vi "Analog Output DAQ Engine.vi"(8 "error in":errorcluster, 10 "DAQ Engine":refnum<notifier>, 11 "Sequence Context In":refnum<k7>) -> (0 "error out":errorcluster)   [LabVIEW 2023, in "LTT_TeststandSteptypes.lvlib"]
uses:
  LTT_TeststandSteptypes.lvlib
  HardwareAbstractionLayer_LVOOP/Main/Class Ref.ctl
  HardwareAbstractionLayer_LVOOP/DMM/DMM.lvclass
  HardwareAbstractionLayer_LVOOP/Function Generator/Function Generator.lvclass
  HardwareAbstractionLayer_LVOOP/Oscilloscope/Oscilloscope.lvclass
  HardwareAbstractionLayer_LVOOP/PowerSupply/PowerSupply.lvclass
  HardwareAbstractionLayer_LVOOP/Teststand/Teststand.lvclass
  HardwareAbstractionLayer_LVOOP/Analog Output/AO/AO.lvclass
  HardwareAbstractionLayer_LVOOP/Analog Input/AI/AI.lvclass
  HardwareAbstractionLayer_LVOOP/Database/Database.lvclass
  HardwareAbstractionLayer_LVOOP/Digital Output/DO_class/DO.lvclass
  HardwareAbstractionLayer_LVOOP/Digital Input/DI_class/DI.lvclass
  HardwareAbstractionLayer_LVOOP/PWM Output/PWM Output_class/PWM Output.lvclass
  HardwareAbstractionLayer_LVOOP/PWM Input/PWM Input_class/PWM Input.lvclass
  HardwareAbstractionLayer_LVOOP/NI Switch/NISwitch_class/NISwitch.lvclass
  HardwareAbstractionLayer_LVOOP/Modbus/Modbus_class/Modbus.lvclass
  HardwareAbstractionLayer_LVOOP/CAN/CAN Lib/CAN_class/CAN.lvclass
  HardwareAbstractionLayer_LVOOP/Analog Output/NI Analog Output/NI Analog Output.lvclass
  D:/eDCU LTT/VT LTT Project/Source Code/HardwareAbstractionLayer_LVOOP/Analog Output/AO/AO.lvclass
  HardwareAbstractionLayer_LVOOP/Main/Class Options.ctl
  <vilib>/Utility/error.llb/DialogType.ctl
  HardwareAbstractionLayer_LVOOP/Main/Main.lvclass
panel:
  in  "stop":bool
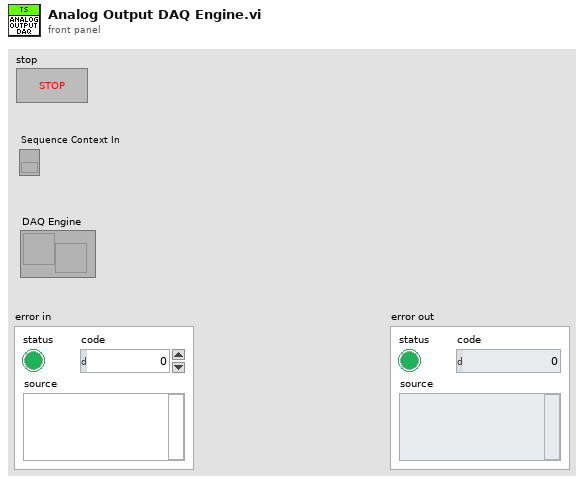
[diagram p1: front panel]
types:
  T1 = typedef "HardwareAbstractionLayer_LVOOP.lvlib/Main.lvclass/Class Ref.ctl" = cluster{"DMM":refnum<class "DMM.lvclass">, "Function Generator":refnum<class "Function Generator.lvclass">, "Oscilloscope":refnum<class "Oscilloscope.lvclass">, "PowerSupply":refnum<class "PowerSupply.lvclass">, "Teststand":refnum<class "Teststand.lvclass">, "AO":refnum<class "AO.lvclass">, "AI":refnum<class "AI.lvclass">, "Database":refnum<class "Database.lvclass">, "AO Waveform Generation":refnum<class "AO.lvclass">, "DO":refnum<class "DO.lvclass">, "DI":refnum<class "DI.lvclass">, "PWM Output":refnum<class "PWM Output.lvclass">, "PWM Input":refnum<class "PWM Input.lvclass">, "RelayOutput":refnum<class "NISwitch.lvclass">, "Modbus":refnum<class "Modbus.lvclass">, "CAN":refnum<class "CAN.lvclass">}
  T2 = typedef "HardwareAbstractionLayer_LVOOP.lvlib/Main.lvclass/Class Options.ctl" = enum16{"Init All Class", "Read All Class", "Write AI Class", "Write AO Class", "Write AO Waveform Generation", "Write DI Class", "Write DO Class", "Write PWM Input Class", "Write PWM Output Class", "Exit"}
  T3 = typedef "DialogType.ctl" = u16
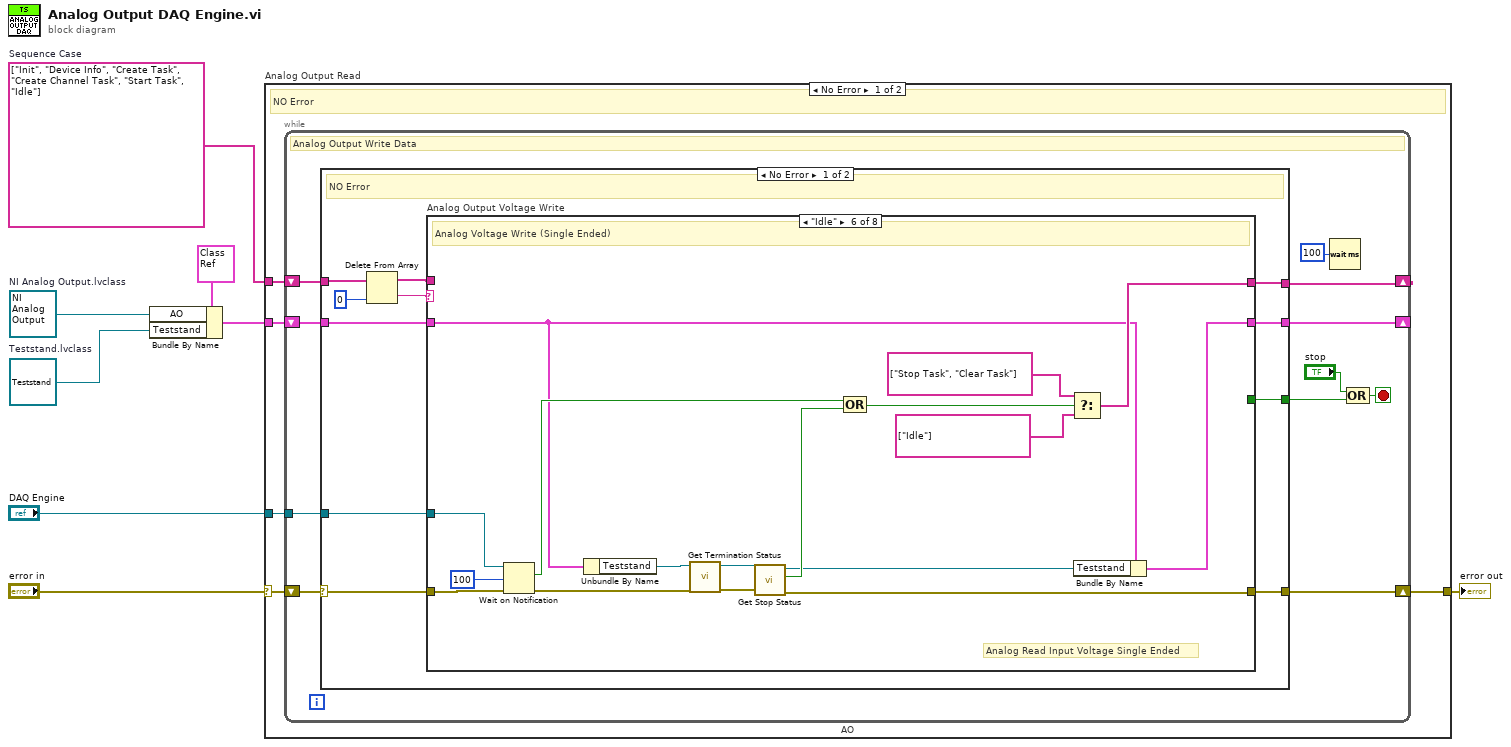
[diagram p0: block diagram]
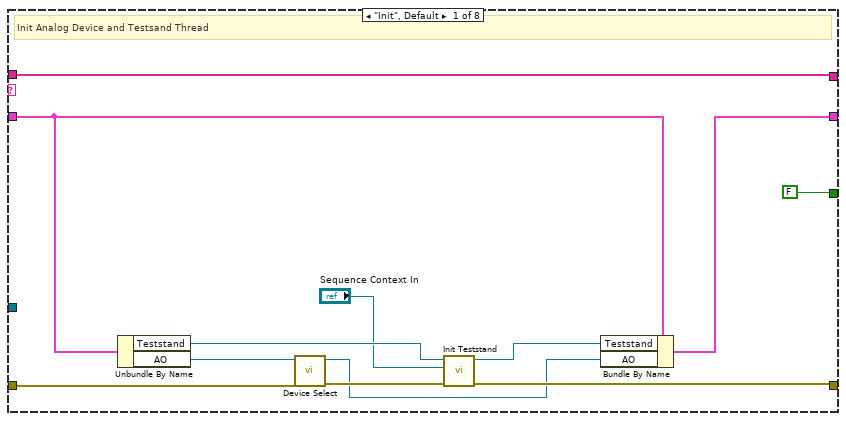
[diagram p2: hidden frame]
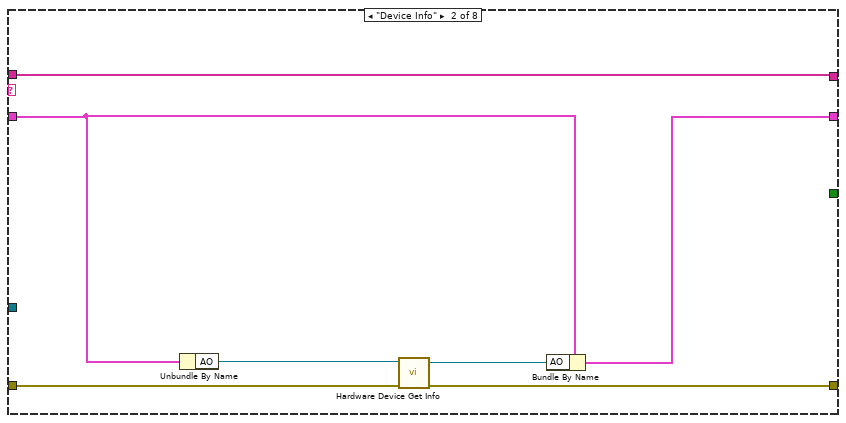
[diagram p3: hidden frame]
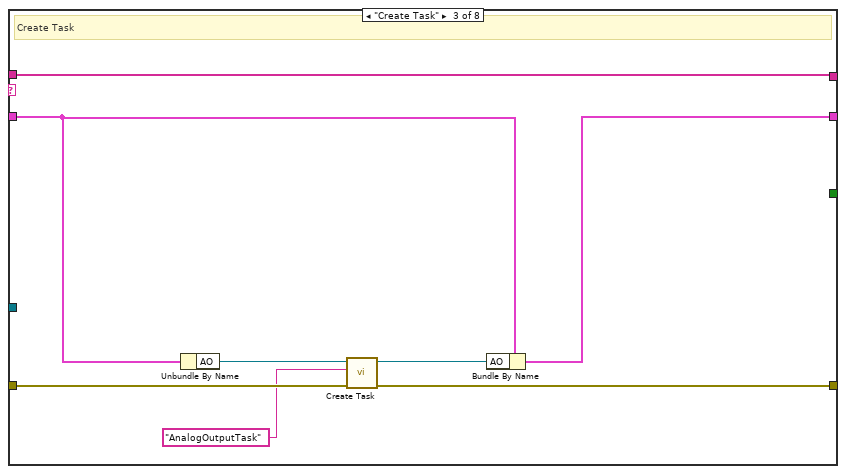
[diagram p4: hidden frame]
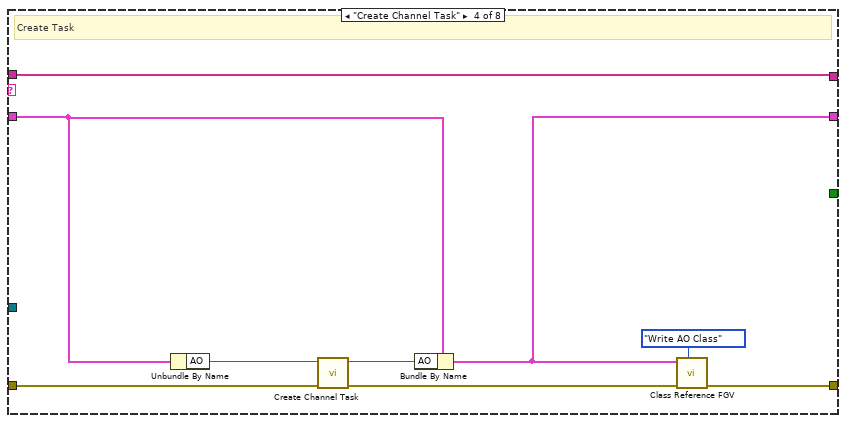
[diagram p5: hidden frame]
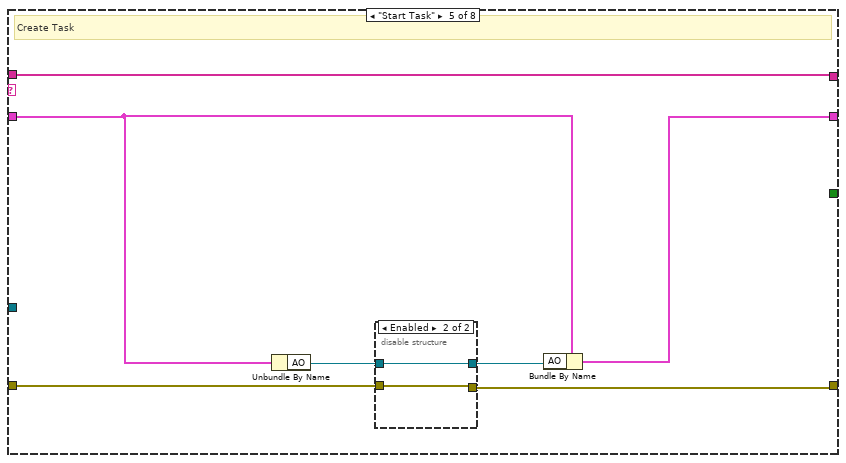
[diagram p6: hidden frame]
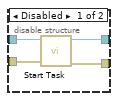
[diagram p7: hidden frame]
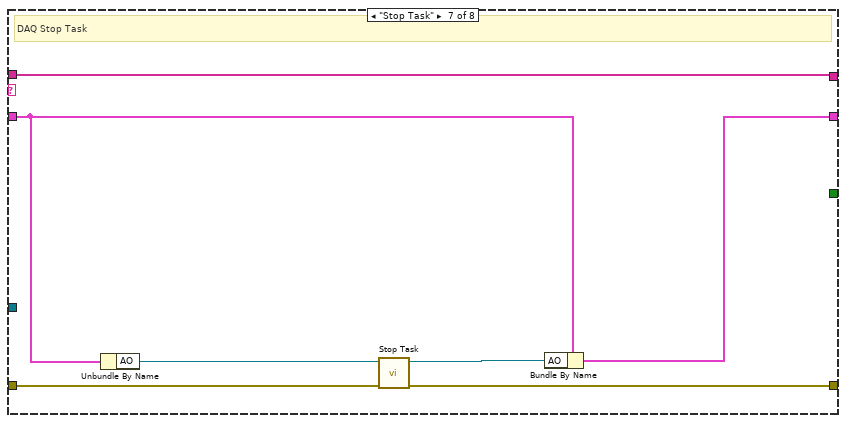
[diagram p8: hidden frame]
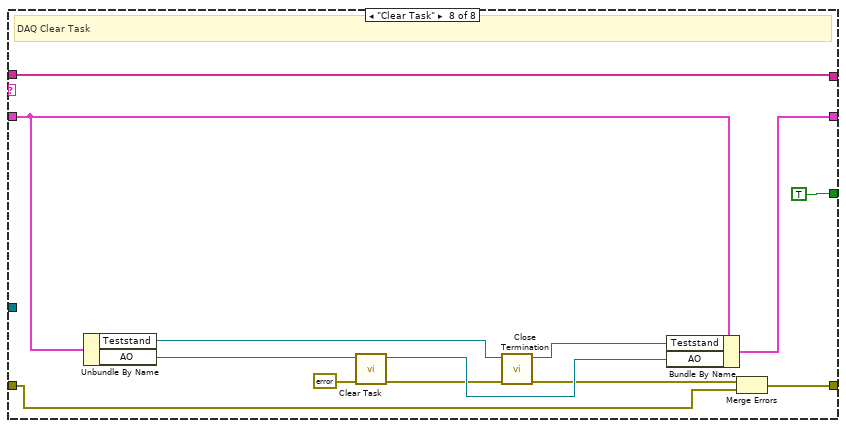
[diagram p9: hidden frame]
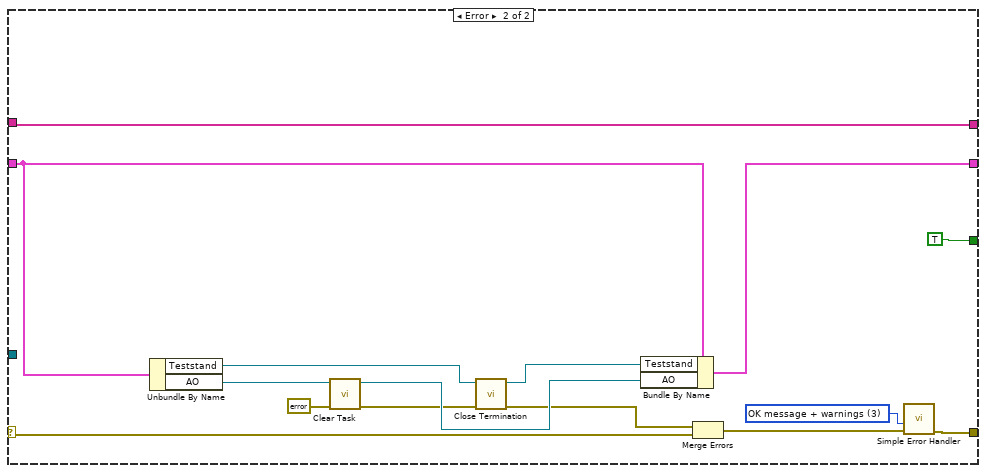
[diagram p10: hidden frame]
diagram:
  w1 = refnum<class "Teststand.lvclass"> refnum  # Teststand.lvclass
  w3 = refnum<class "NI Analog Output.lvclass"> refnum  # NI Analog Output.lvclass
  w4 = string[] ["Init", "Device Info", "Create Task", "Create Channel Task", "Start Task", "Idle"]  # Sequence Case
  n1 = Bundle By Name(cluster=T1 {"DMM"=refnum, "Function Generator"=refnum, "Oscilloscope"=refnum, "PowerSupply"=refnum, "Teststand"=refnum, "AO"=refnum, "AI"=refnum, "Database"=refnum, "AO Waveform Generation"=refnum, "DO"=refnum, "DI"=refnum, "PWM Output"=refnum, "PWM Input"=refnum, "RelayOutput"=refnum, "Modbus"=refnum, "CAN"=refnum} ("Class Cluster"), "AO"=w3, "Teststand"=w1) -> (w5:T1)
  n2 = case "Analog Output Read" shown="No Error" "error in" {
    selector: "error in" -> [w13 w137]
    tunnel: [w12 w137] -> w7
    tunnel: w5 -> [w11 _]
    tunnel: w4 -> [w10 _]
    tunnel: "DAQ Engine" -> [w9 _]
    frame No Error {
      # "NO Error"
      n3 = while "AO" {
        shift-right: [w23] -> w12
        shift-left: w13 -> [w24]
        shift-right: [w21] -> _
        shift-left: w11 -> [w22]
        shift-right: [w19] -> _
        shift-left: w10 -> [w20]
        tunnel: w9 -> [w14]
        stop <- w16 stop-if-true
        # "Analog Output Write Data"
        n4 = case shown="No Error" w24 {
          selector: w24 -> [w35 w128]
          tunnel: [w34 w123] -> w23
          tunnel: w22 -> [w30 w126]
          tunnel: [w29 w127] -> w21
          tunnel: w20 -> [w33 w125]
          tunnel: [w27 w125] -> w19
          tunnel: [w26 TRUE] -> w15
          tunnel: w14 -> [w25 _]
          frame No Error {
            # "NO Error"
            n5 = Delete From Array(array=w33, index=0) -> (deleted portion=w32:string, array with subset deleted=w28:string[])  [unwired: 1 in]
            n6 = case "Analog Output Voltage Write" shown="\"Idle\"" w32 {
              tunnel: w35 -> [w43 w51 w59 w69 w75 w101 w105 w109]
              tunnel: [w38 w50 w58 w65 w73 w89 w104 w110] -> w34
              tunnel: w30 -> [w46 w53 w61 w70 w77 w87 w107 w120]
              tunnel: [w45 w52 w60 w63 w76 w86 w106 w119] -> w29
              tunnel: w28 -> [w47 w54 w62 w71 w78 _ w108 w121]
              tunnel: [w47 w54 w62 w71 w78 w98 w108 w121] -> w27
              tunnel: [FALSE _ _ _ _ _ _ TRUE] -> w26
              tunnel: w25 -> [_ _ _ _ _ w96 _ _]
              frame "Init", Default {
                # "Init Analog Device and Testsand Thread"
                n7 = Unbundle By Name(w46) -> ("Teststand"=w41:refnum<class "Teststand.lvclass">, "AO"=w42:refnum<class "AO.lvclass">)
                n8 = call-dynamic "Device Select.vi"("error in (no error)"=w43, "AO in"=w42) -> ("error out"=w39:errorcluster, "AO out"=w36:refnum<class "AO.lvclass">)  [unwired: 8 in]
                n9 = call-dynamic "Init Teststand.vi"("error in (no error)"=w39, "Sequence Context In"="Sequence Context In", "Teststand in"=w41) -> ("error out"=w38:errorcluster, "Teststand out"=w37:refnum<class "Teststand.lvclass">)  [unwired: 7 in]
                n10 = Bundle By Name(cluster=w46, "Teststand"=w37, "AO"=w36) -> (w45:T1)
              }
              frame "Device Info" {
                n11 = Unbundle By Name(w53) -> ("AO"=w48:refnum<class "AO.lvclass">)
                n12 = call-dynamic "Hardware Device Get Info.vi"("error in (no error)"=w51, "AO in"=w48) -> ("error out"=w50:errorcluster, "AO out"=w49:refnum<class "AO.lvclass">)  [unwired: 8 in]
                n13 = Bundle By Name(cluster=w53, "AO"=w49) -> (w52:T1)
              }
              frame "Create Task" {
                # "Create Task"
                n14 = Unbundle By Name(w61) -> ("AO"=w56:refnum<class "AO.lvclass">)
                n15 = call-dynamic "Create Task.vi"("error in (no error)"=w59, "Task name"="AnalogOutputTask", "AO in"=w56) -> ("error out"=w58:errorcluster, "AO out"=w57:refnum<class "AO.lvclass">)  [unwired: 7 in]
                n16 = Bundle By Name(cluster=w61, "AO"=w57) -> (w60:T1)
              }
              frame "Create Channel Task" {
                # "Create Task"
                n17 = Unbundle By Name(w70) -> ("AO"=w67:refnum<class "AO.lvclass">)
                n18 = call-dynamic "Create Channel Task.vi"("error in (no error)"=w69, "AO in"=w67) -> ("error out"=w66:errorcluster, "AO out"=w68:refnum<class "AO.lvclass">)  [unwired: 8 in]
                n19 = Bundle By Name(cluster=w70, "AO"=w68) -> (w63:T1)
                n20 = call "Class Reference FGV.vi"("Options"=Class_Options."Write AO Class", "error in"=w66, "Class Cluster In"=w63) -> ("error out"=w65:errorcluster)  [unwired: 7 in, 1 out]
              }
              frame "Start Task" {
                # "Create Task"
                n21 = Unbundle By Name(w77) -> ("AO"=w74:refnum<class "AO.lvclass">)
                n22 = disable-structure shown="Enabled" {
                  disable-tunnel: w75 -> [w82 w83]
                  disable-tunnel: w74 -> [w81 w84]
                  disable-tunnel: [w80 w83] -> w73
                  disable-tunnel: [w79 w84] -> w72
                  frame Disabled {
                    n23 = call-dynamic "Start Task.vi"("error in (no error)"=w82, "AO in"=w81) -> ("error out"=w80:errorcluster, "AO out"=w79:refnum<class "AO.lvclass">)  [unwired: 8 in]
                  }
                  frame Enabled {
                  }
                }
                n24 = Bundle By Name(cluster=w77, "AO"=w72) -> (w76:T1)
              }
              frame "Idle" {
                # "Analog Read Input Voltage Single Ended"
                # "Analog Voltage Write (Single Ended)"
                n25 = Wait on Notification(notifier=w96, timeout in ms (-1)=100, error in (no error)=w101) -> (notification=w94:bool, error out=w91:errorcluster)  [unwired: 1 in, 2 out]
                n26 = Unbundle By Name(w87) -> ("Teststand"=w93:refnum<class "Teststand.lvclass">)
                n27 = call-dynamic "Get Termination Status.vi"("error in (no error)"=w91, "Teststand in"=w93) -> ("error out"=w90:errorcluster, "Teststand out"=w92:refnum<class "Teststand.lvclass">)  [unwired: 7 in, 1 out]
                n28 = call-dynamic "Get Stop Status.vi"("error in (no error)"=w90, "Teststand in"=w92) -> ("error out"=w89:errorcluster, "Value"=w88:bool, "Teststand out"=w85:refnum<class "Teststand.lvclass">)  [unwired: 7 in]
                n29 = Compound Arithmetic op=OR(w94, w88) -> (w97:bool)
                n30 = Select(t=string[] ["Stop Task", "Clear Task"], s=w97, f=string[] ["Idle"]) -> (s? t:f=w98:string[])
                n31 = Bundle By Name(cluster=w87, "Teststand"=w85) -> (w86:T1)
              }
              frame "Stop Task" {
                # "DAQ Stop Task"
                n32 = Unbundle By Name(w107) -> ("AO"=w102:refnum<class "AO.lvclass">)
                n33 = call-dynamic "Stop Task.vi"("error in (no error)"=w105, "AO in"=w102) -> ("error out"=w104:errorcluster, "AO out"=w103:refnum<class "AO.lvclass">)  [unwired: 8 in]
                n34 = Bundle By Name(cluster=w107, "AO"=w103) -> (w106:T1)
              }
              frame "Clear Task" {
                # "DAQ Clear Task"
                n35 = Unbundle By Name(w120) -> ("Teststand"=w115:refnum<class "Teststand.lvclass">, "AO"=w117:refnum<class "AO.lvclass">)
                n36 = call-dynamic "Clear Task.vi"("error in (no error)"=errorcluster {"status"=FALSE, "code"=0, "source"=""}, "AO in"=w117) -> ("error out"=w114:errorcluster, "AO out"=w116:refnum<class "AO.lvclass">)  [unwired: 8 in]
                n37 = call-dynamic "Close Termination.vi"("error in (no error)"=w114, "Teststand in"=w115) -> ("error out"=w112:errorcluster, "Teststand out"=w113:refnum<class "Teststand.lvclass">)  [unwired: 8 in]
                n38 = Bundle By Name(cluster=w120, "Teststand"=w113, "AO"=w116) -> (w119:T1)
                n39 = Merge Errors(w112, w109) -> (w110:errorcluster)
              }
            }
          }
          frame Error {
            w122 = T3 3 items=["no dialog", "OK message", "continue or stop message", "OK message + warnings", "continue/stop + warnings"] ("type of dialog (OK msg:1)")
            n40 = Unbundle By Name(w126) -> ("Teststand"=w133:refnum<class "Teststand.lvclass">, "AO"=w135:refnum<class "AO.lvclass">)
            n41 = call-dynamic "Clear Task.vi"("error in (no error)"=errorcluster {"status"=FALSE, "code"=0, "source"=""}, "AO in"=w135) -> ("error out"=w132:errorcluster, "AO out"=w134:refnum<class "AO.lvclass">)  [unwired: 8 in]
            n42 = call-dynamic "Close Termination.vi"("error in (no error)"=w132, "Teststand in"=w133) -> ("error out"=w130:errorcluster, "Teststand out"=w131:refnum<class "Teststand.lvclass">)  [unwired: 8 in]
            n43 = Bundle By Name(cluster=w126, "Teststand"=w131, "AO"=w134) -> (w127:T1)
            n44 = Merge Errors(w130, w128) -> (w124:errorcluster)
            n45 = call <vilib>:"Simple Error Handler.vi"("type of dialog (OK msg:1)"=w122, "error in (no error)"=w124) -> ("error out"=w123:errorcluster)  [unwired: 3 in, 4 out]
          }
        }
        n46 = Wait (ms)(milliseconds to wait=u32 100) -> ()  [unwired: 1 out]
        n47 = Compound Arithmetic op=OR("stop", w15) -> (w16:bool)
      }
    }
    frame Error {
      # "Error"
    }
  }
  "error out" <- w7
